vi "RenderLine.vi"(4 "y2":sgl, 6 "x2":sgl, 8 "No Error":errorcluster, 9 "y1":sgl, 10 "x1":sgl, 11 "Renderer [SDL_Renderer *]":T1 format="%.0x") -> (0 "error out":errorcluster)   [LabVIEW 2026, in "SDL3.lvlib" / "Render.lvlib"]
doc: "<B>Summary</B>\nDraw a line on the current rendering target at subpixel precision."
uses:
  Render.lvlib
  <vilib>/Utility/error.llb/Error Cluster From Error Code.vi
  Error/Error.lvlib
  Lib/SDL3.dll
  SDL_Renderer--pointer.ctl
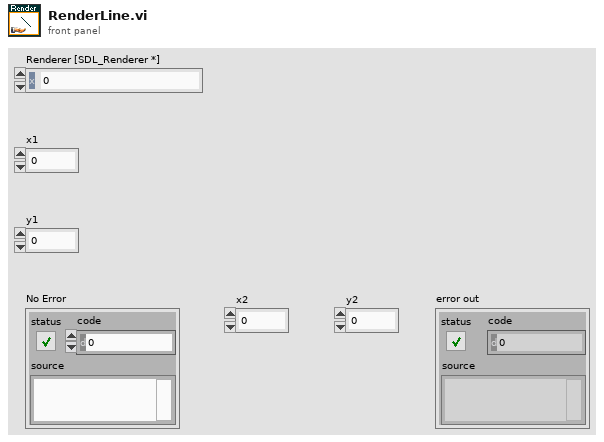
[diagram p1: front panel]
types:
  T1 = typedef "SDL3.lvlib/Render.lvlib/SDL_Renderer--pointer.ctl" = i64
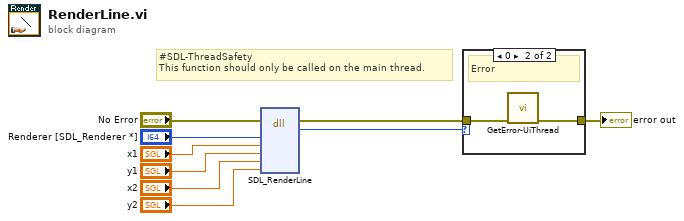
[diagram p0: block diagram]
diagram:
  # "#SDL-ThreadSafety\nThis function should only be called on the main thread."
  n1 = dll-call lib="C:/Users/saukko/Dev/LV-SDL3/Sources/SDL3/Lib/SDL3.*" fn="SDL_RenderLine"(error in="No Error", "renderer"="Renderer [SDL_Renderer *]", "x1"="x1", "y1"="y1", "x2"="x2", "y2"="y2") -> (error out=w2:errorcluster, "return type"=w1:i32)  [unwired: 7 in, 1 out]
  n2 = case shown="0" w1 {
    tunnel: w2 -> [w10 w12]
    tunnel: [w10 w11] -> w8
    frame Default {
      # "Ok"
    }
    frame 0 {
      # "Error"
      n3 = call "GetError-UiThread.vi"("No Error"=w12) -> ("error out"=w11:errorcluster)  [unwired: 10 in]
    }
  }
  "error out" <- w8
